vi "Alp Proj Control Ex.vi"(8 "error in (no error)":errorcluster, 9 "pUserStructPtr":u32, 10 "ControlType":i32, 11 "DeviceId":u32) -> (0 "error out":errorcluster, 1 "pUserStructPtr out":u32, 3 "function return":i32)   [LabVIEW 2013, in "alpD41.lvlib"]
uses:
  <userlib>/alpD41/alpD41.lvlib
  <userlib>/alpD41/alpD41.dll
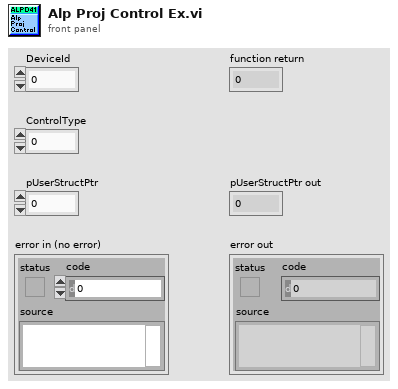
[diagram p1: front panel]
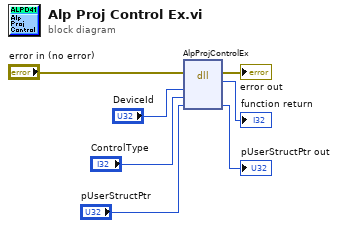
[diagram p0: block diagram]
diagram:
  n1 = dll-call lib="C:/Program Files (x86)/National Instruments/LabVIEW 2013/user.lib/alpD41/alpD41.*" fn="AlpProjControlEx"(error in="error in (no error)", "DeviceId"="DeviceId", "ControlType"="ControlType", "pUserStructPtr"="pUserStructPtr") -> (error out=→"error out":errorcluster, →"function return":i32, "pUserStructPtr"=→"pUserStructPtr out":u32)  [unwired: 4 in, 1 out]
